vi "Test_getEvent_softwareVersions.vi"(8 "error in (no error)":errorcluster, 11 "logevent_softwareVersions_Ctl":T1={"private_rcvStamp"=0.0, "salVersion"="                                                                                                                                                                                                                                                                ", "xmlVersion"="", "openSpliceVersion"="                                                                                                                                                                                                                                                                ", "cscVersion"="", "subsystemVersions"="", "priority"=0}) -> (0 "error out":errorcluster, 2 "function return":i32, 3 "logevent_softwareVersions_Ctl out":T1={"private_rcvStamp"=0.0, "salVersion"="                                                                                                                                                                                                                                                                ", "xmlVersion"="", "openSpliceVersion"="                                                                                                                                                                                                                                                                ", "cscVersion"="", "subsystemVersions"="", "priority"=0})   [LabVIEW 2018, in "SALLV_Test.lvlib"]
doc: "int Test_shm_getEvent_softwareVersionsLV(Test_logevent_softwareVersionsLV *logevent_softwareVersions_Ctl );"
uses:
  DataTypes/logevent_softwareVersions.ctl
  SALLV_Test.lvlib
  SALLV_Test.so
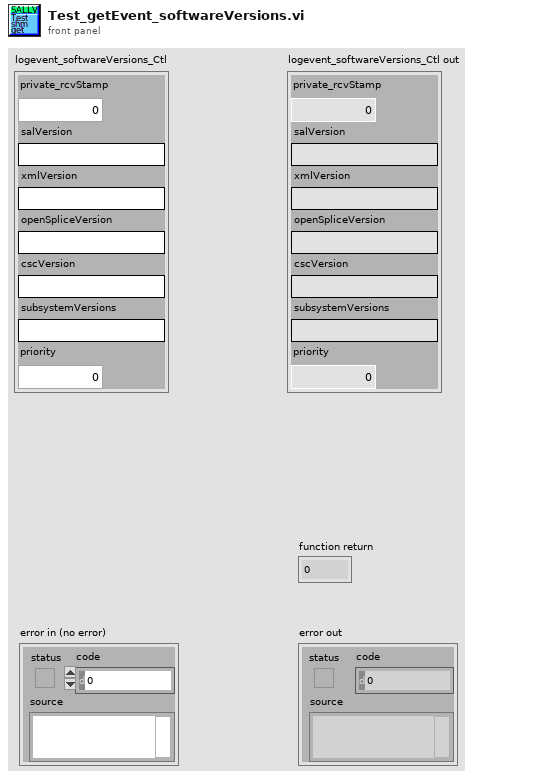
[diagram p1: front panel]
types:
  T1 = typedef "SALLV_Test.lvlib/logevent_softwareVersions.ctl" = cluster{"private_rcvStamp":dbl, "salVersion":string, "xmlVersion":string, "openSpliceVersion":string, "cscVersion":string, "subsystemVersions":string, "priority":i32}
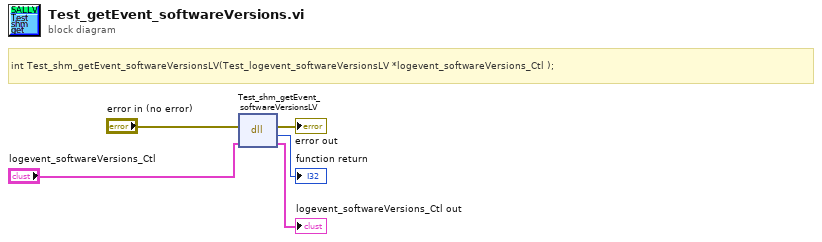
[diagram p0: block diagram]
diagram:
  # "int Test_shm_getEvent_softwareVersionsLV(Test_logevent_softwareVersionsLV *logevent_softwareVersions_Ctl );"
  n1 = dll-call lib="home/ttsai/Documents/salTestLabViewApi/SALLV_Test/SALLV_Test.*" fn="Test_shm_getEvent_softwareVersionsLV"(error in="error in (no error)", "logevent_softwareVersions_Ctl"="logevent_softwareVersions_Ctl") -> (error out=→"error out":errorcluster, →"function return":i32, "logevent_softwareVersions_Ctl"=→"logevent_softwareVersions_Ctl out":T1)  [unwired: 2 in, 1 out]
